vi "Teleop.vi"(10 "Match Info":T1={"Autonomous Elapsed Seconds"=0.0, "TeleOp Elapsed Seconds"=0.0, "Disabled Elapsed Seconds"=0.0, "Visited Autonomous"=FALSE, "Visited TeleOp"=FALSE, "Visited Disabled"=FALSE, "Autonomous Settings"={"Autonomous Style"=enum."Independent", "VI Refnum"=refnum}}, 11 "Call Context":T2) -> ()   [LabVIEW 2019]
doc: "This VI is called for each TeleOp packet received from the DS where the robot is not disabled. It is often used to read from the joysticks and update I/O or to update setpoints for timed control loops. It should complete and return within 20 milliseconds or it may miss DS packets."
uses:
  <vilib>/Rock Robotics/Network Tables/NT Write Numeric Array.vi
  Robot Global Data.vi
  <vilib>/Rock Robotics/Network Tables/NT Write Number.vi
  <vilib>/Rock Robotics/Network Tables/NT Write Variant.vi
  <vilib>/Rock Robotics/Network Tables/NT Write Boolean.vi
  <vilib>/Rock Robotics/Network Tables/NT Write Boolean Array.vi
  <vilib>/Rock Robotics/Network Tables/NT Write String.vi
  <vilib>/Rock Robotics/WPI/DriverStation/WPI_DriverStationMatch Info.ctl
  <vilib>/Rock Robotics/WPI/DriverStation/WPI_DriverStationDerivedRobotMode.ctl
panel:
  in  "Blue Cal":cluster{"R":dbl, "G":dbl, "B":dbl}={"R"=0.143, "G"=0.427, "B"=0.429} caption="Blue Calibration"
  in  "Green Cal":cluster{"R":dbl, "G":dbl, "B":dbl}={"R"=0.197, "G"=0.561, "B"=0.24} caption="Green Calibration"
  in  "Red Cal":cluster{"R":dbl, "G":dbl, "B":dbl}={"R"=0.561, "G"=0.323, "B"=0.114} caption="Red Calibration"
  in  "Yellow Cal":cluster{"R":dbl, "G":dbl, "B":dbl}={"R"=0.361, "G"=0.524, "B"=0.113} caption="Yellow Calibration"
  out "Matched Color Name":string
  out "Match Confidence":dbl
  out "Measured Color":cluster{"R":dbl, "G":dbl, "B":dbl}
  out "error out 2":errorcluster
  out "Proximity":u16(graph)
  out "Color":u32(colorbox)
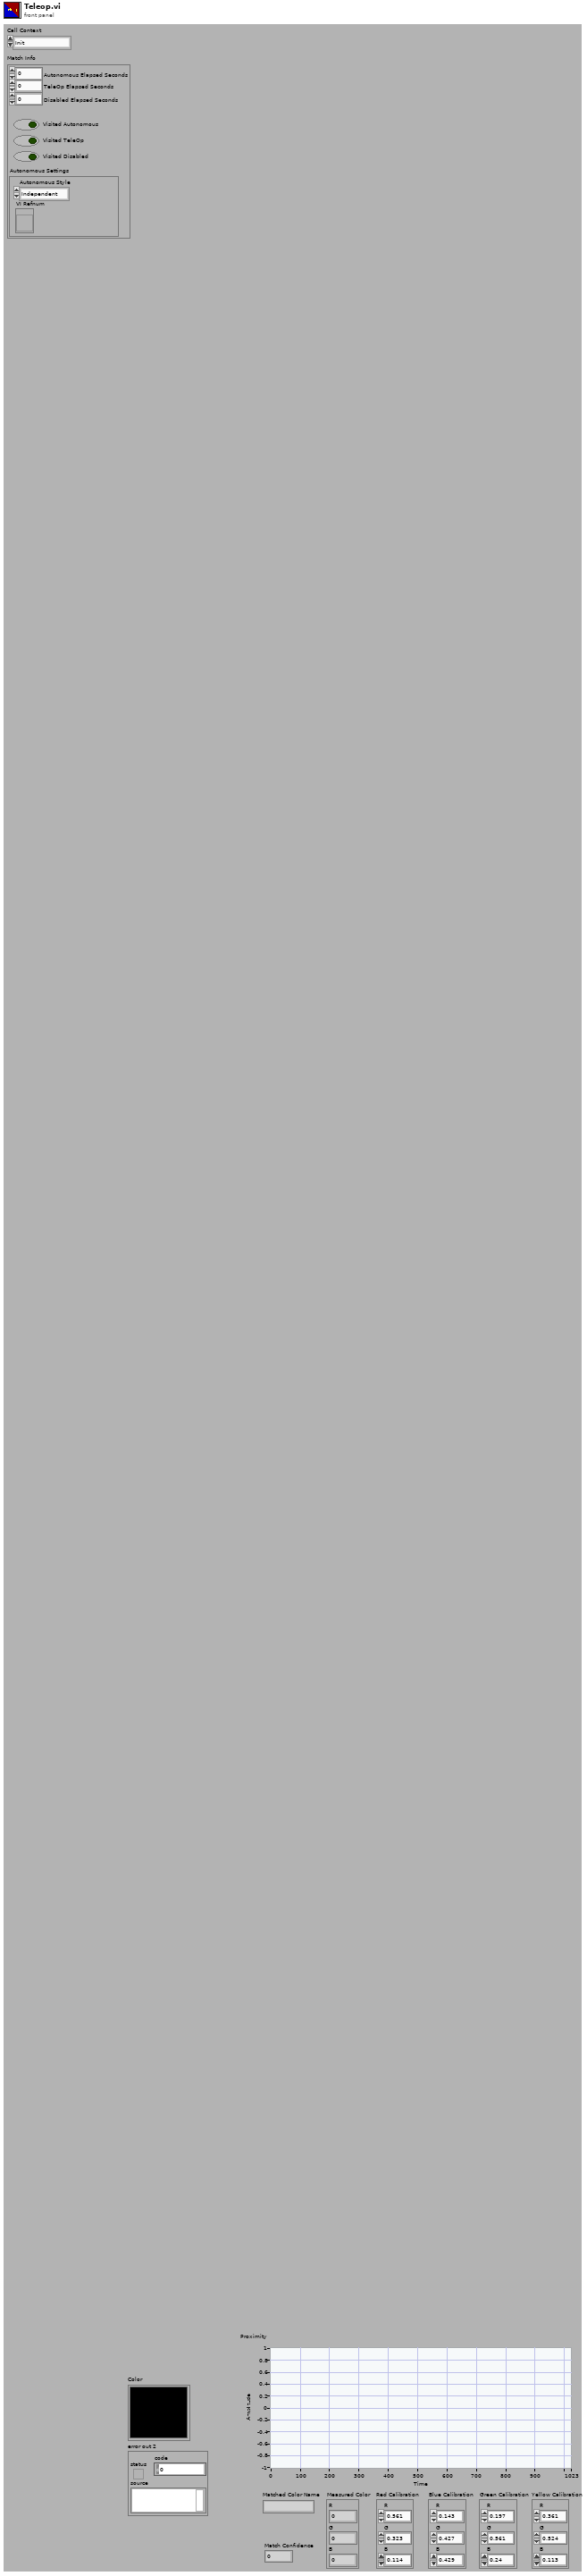
[diagram p1: front panel]
types:
  T1 = typedef "WPI_DriverStationMatch Info.ctl" = cluster{"Autonomous Elapsed Seconds":dbl, "TeleOp Elapsed Seconds":dbl, "Disabled Elapsed Seconds":dbl, "Visited Autonomous":bool, "Visited TeleOp":bool, "Visited Disabled":bool, "Autonomous Settings":cluster{"Autonomous Style":enum16{"Iterative", "Independent"}, "VI Refnum":refnum<vi>}}
  T2 = typedef "WPI_DriverStationDerivedRobotMode.ctl" = enum16{"Init", "Execute", "Stop"}
  T3 = typedef "WPI_RobotDriveDevRef.ctl" = cluster{"DevStatus":errorcluster, "Motors[]":T4[], "Square Inputs":bool, "Max Output":dbl}
  T4 = typedef "WPI_MotorControlDeviceRef.ctl" = cluster{"DeviceStatus":errorcluster, "Type":T5, "PWM":cluster{"PWM Channel":T6, "DeadBand":T7}, "CAN":cluster{"Device Number":u8, "SetOutput VI Ref":variant, "GetOutput VI Ref":variant, "Enable VI Ref":variant, "Disable VI Ref":variant, "Data":variant}, "Invert":bool, "DIO PWM":cluster{"PWM \"Enable\" Channel":T6, "DIOChannel":T8, "PWM Rate":dbl}}
  T5 = typedef "WPI_MotorControlType.ctl" = enum16{"PWM", "CAN", "DIO PWM"}
  T6 = typedef "FPGA_DIOPWMChannel.ctl" = enum8{"PWM 0", "PWM 1", "PWM 2", "PWM 3", "PWM 4", "PWM 5", "PWM 6", "PWM 7", "PWM 8", "PWM 9", "PWM MXP 0", "PWM MXP 1", "PWM MXP 2", "PWM MXP 3", "PWM MXP 4", "PWM MXP 5", "PWM MXP 6", "PWM MXP 7", "PWM MXP 8", "PWM MXP 9", "Invalid"}
  T7 = typedef "WPI_PWMDeadband.ctl" = cluster{"Name":string, "maxPositivePwm":i32, "minPositivePwm":i32, "centerPwm":i32, "maxNegativePwm":i32, "minNegativePwm":i32, "angularRange":u16}
  T8 = typedef "FPGA_DIOChannel.ctl" = enum8{"DIO 0", "DIO 1", "DIO 2", "DIO 3", "DIO 4", "DIO 5", "DIO 6", "DIO 7", "DIO 8", "DIO 9", "DIO MXP 0", "DIO MXP 1", "DIO MXP 2", "DIO MXP 3", "DIO MXP 4", "DIO MXP 5", "DIO MXP 6", "DIO MXP 7", "DIO MXP 8", "DIO MXP 9", "DIO MXP 10", "DIO MXP 11", "DIO MXP 12", "DIO MXP 13", "DIO MXP 14", "DIO MXP 15", "SPI Port CS1", "SPI Port CS2", "SPI Port CS3", "SPI Port MISO", "SPI Port MOSI", "Invalid"}
  T9 = typedef "WPI_JoystickDevRef.ctl" = cluster{"Device":T10}
  T10 = typedef "WPI_JoystickDeviceEnum.ctl" = enum16{"USB 0", "USB 1", "USB 2", "USB 3", "USB 4", "USB 5"}
  T11 = cluster{"JoystickDevRef":T9, "RobotDriveDevRef":T3}
  T12 = typedef "WPI_SwitchDevRef.ctl" = cluster{"DevStatus":errorcluster, "DIO Channel":T8, "CntIndex":T13, "Normally Closed":bool}
  T13 = typedef "FPGA_CounterCtrSystemIndex.ctl" = enum8{"Ctr 0", "Ctr 1", "Ctr 2", "Ctr 3", "Ctr 4", "Ctr 5", "Ctr 6", "Ctr 7", "Invalid"}
  T14 = typedef "Color Sensor V3 DevRef.ctl" = cluster{"I2CDevRef":T15}
  T15 = typedef "WPI_I2CDevRef.ctl" = cluster{"DevStatus":errorcluster, "Device Address":u8, "Handle":i32, "I2C Bus":T16}
  T16 = typedef "i2c_bus.ctl" = enum16{"I2C On-Board", "I2C MXP", "Invalid"}
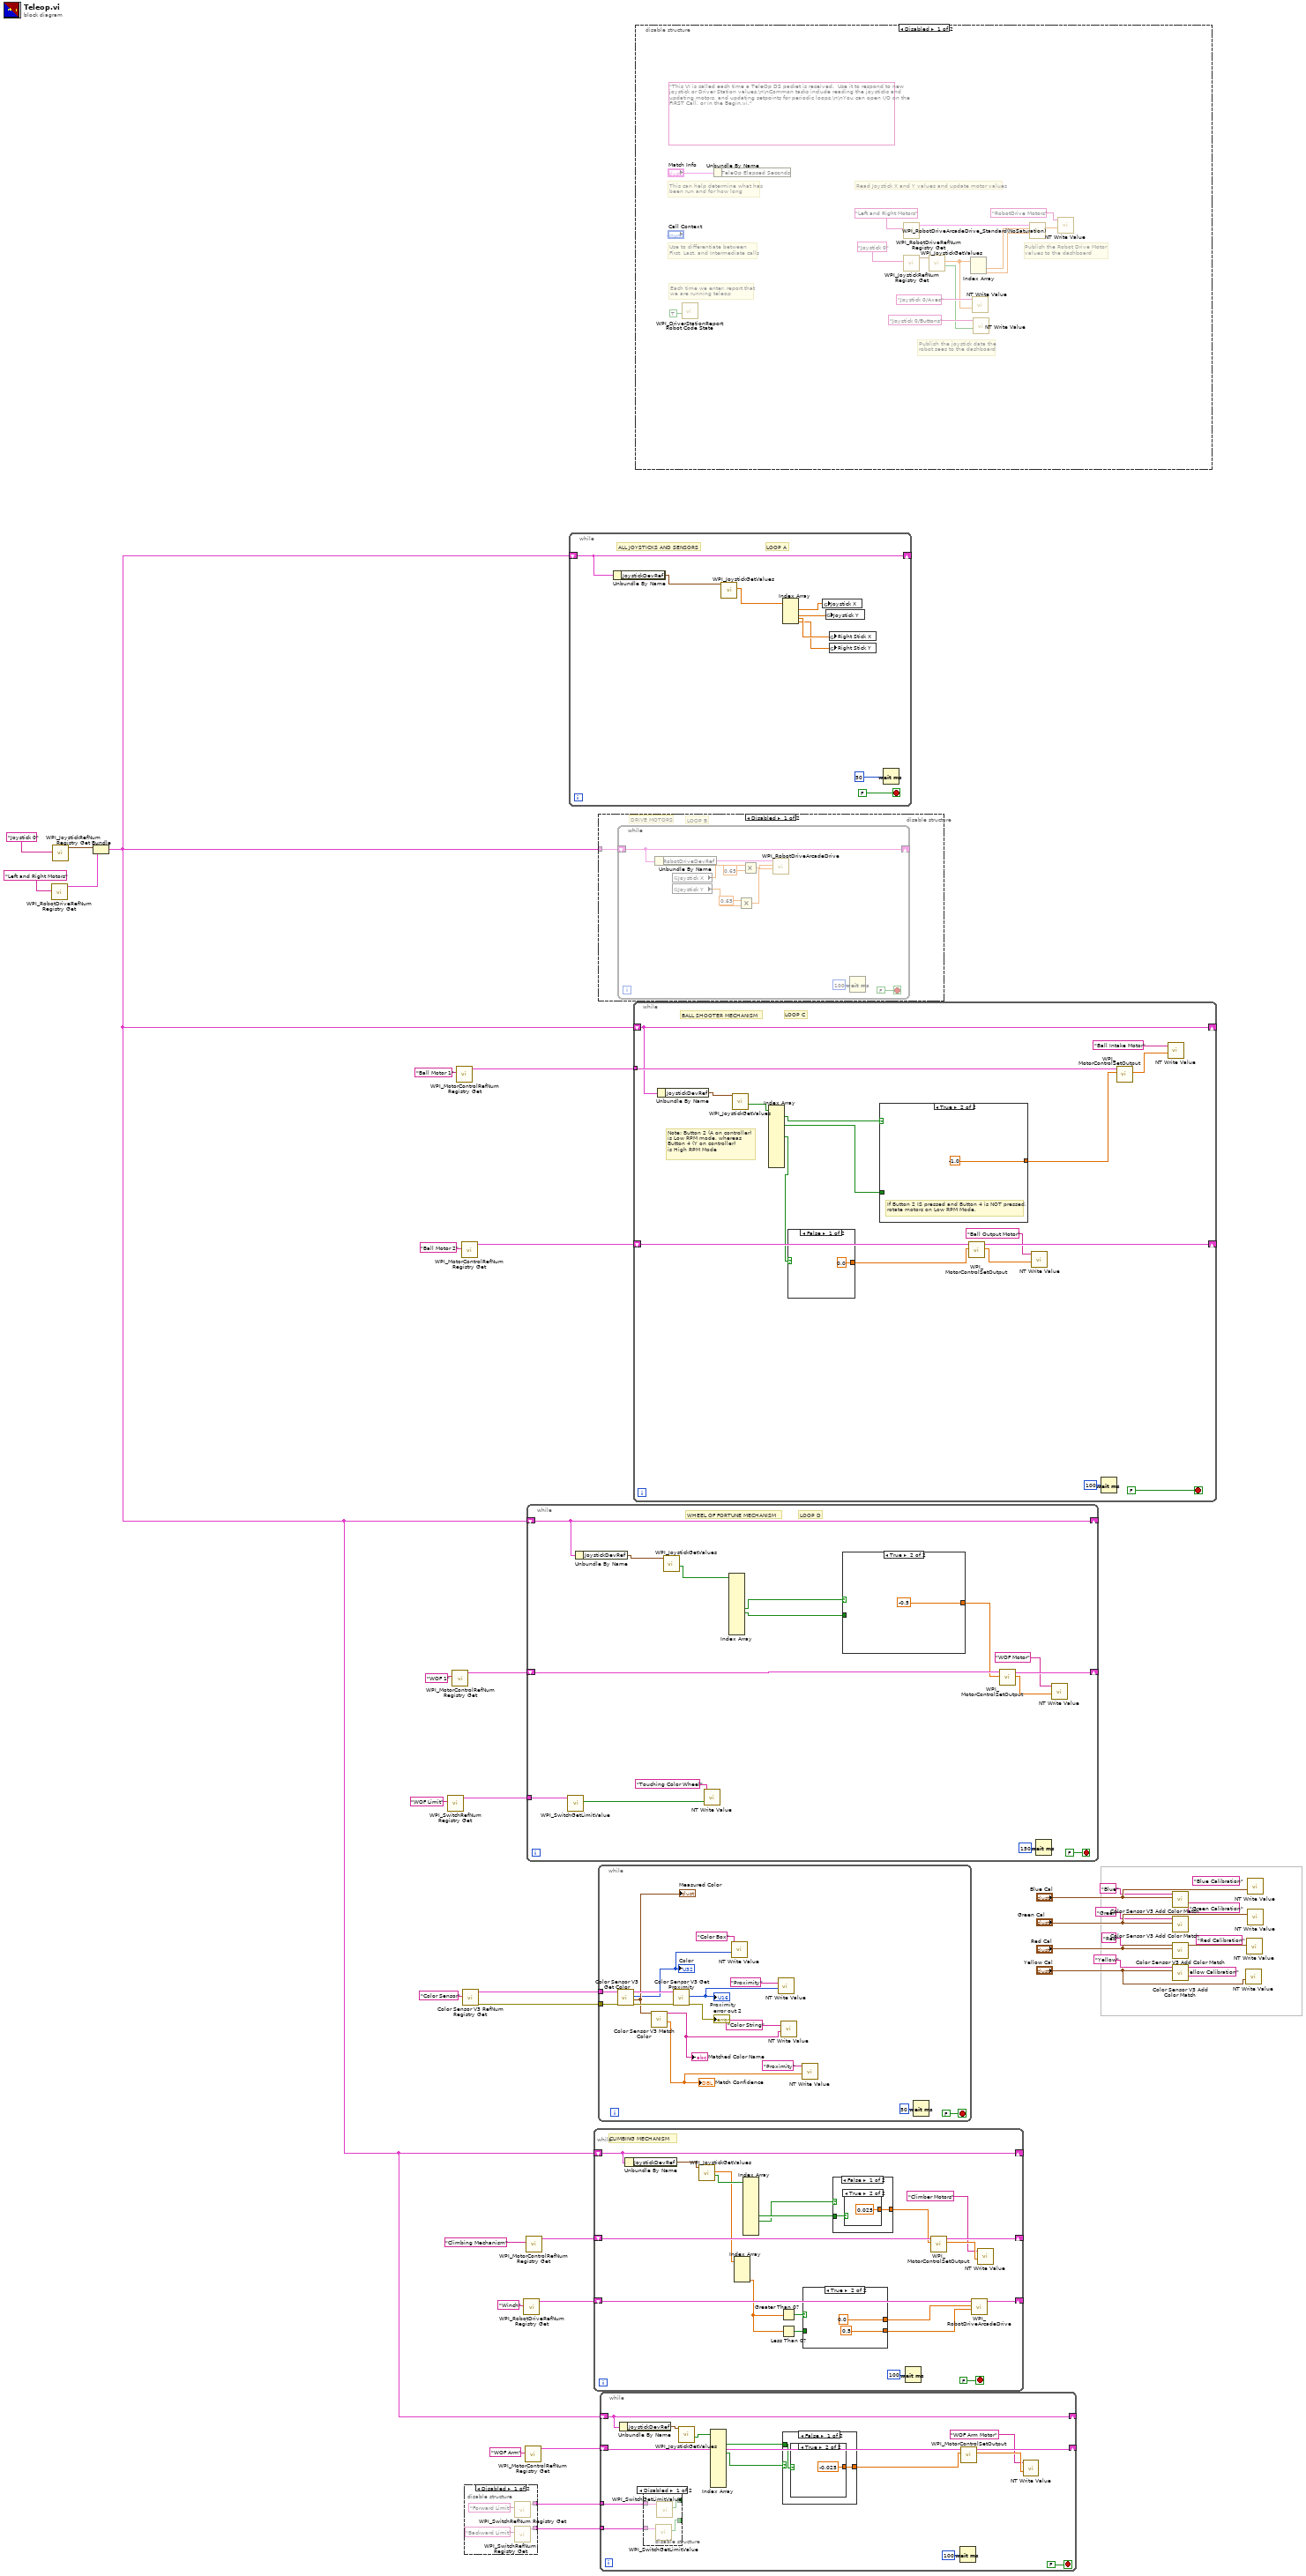
[diagram p0: block diagram]
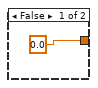
[diagram p3: hidden frame]
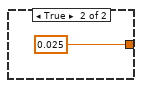
[diagram p4: hidden frame]
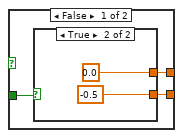
[diagram p6: hidden frame]
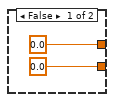
[diagram p7: hidden frame]
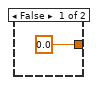
[diagram p8: hidden frame]
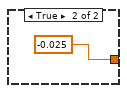
[diagram p9: hidden frame]
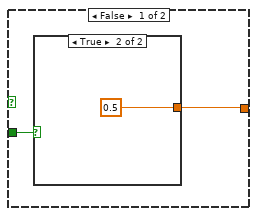
[diagram p12: hidden frame]
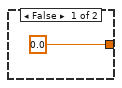
[diagram p13: hidden frame]
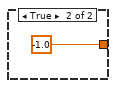
[diagram p14: hidden frame]
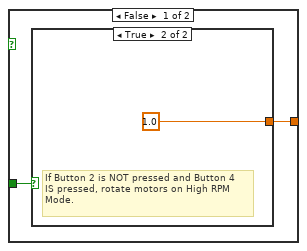
[diagram p15: hidden frame]
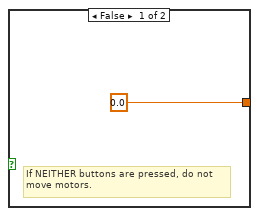
[diagram p16: hidden frame]
diagram:
  (unwired) "Yellow Calibration" ("Name")
  (unwired) "Red Calibration" ("Name")
  (unwired) "Green Calibration" ("Name")
  (unwired) "Blue Calibration" ("Name")
  n1 = call <vilib>:"WPI_RobotDriveRefNum Registry Get.vi"("refnum name"="Left and Right Motors") -> ("RobotDriveDevRef"=w29:T3)  [unwired: 1 in, 9 out]
  n2 = call <vilib>:"WPI_JoystickRefNum Registry Get.vi"("refnum name"="Joystick 0") -> ("JoystickDevRef"=w30:T9)  [unwired: 1 in, 9 out]
  n3 = Bundle("JoystickDevRef"=w30, "RobotDriveDevRef"=w29) -> (w5:T11)  [unwired: 1 out]
  n4 = call <vilib>:"WPI_SwitchRefNum Registry Get.vi"("refnum name"="WOF Limit") -> ("SwitchDevRef"=w10:T12)  [unwired: 9 in, 1 out]
  n5 = call <vilib>:"WPI_MotorControlRefNum Registry Get.vi"("refnum name"="WOF 1") -> ("MotorControlDevRef"=w25:T4)  [unwired: 9 in, 1 out]
  n6 = call <vilib>:"WPI_MotorControlRefNum Registry Get.vi"("refnum name"="Ball Motor 1") -> ("MotorControlDevRef"=w27:T4)  [unwired: 9 in, 1 out]
  n7 = call <vilib>:"WPI_MotorControlRefNum Registry Get.vi"("refnum name"="Ball Motor 2") -> ("MotorControlDevRef"=w12:T4)  [unwired: 9 in, 1 out]
  n8 = call <vilib>:"Color Sensor V3 RefNum Registry Get.vi"("refnum name"="Color Sensor") -> ("error out"=w15:errorcluster, "ColorSensorDevRef"=w16:T14)  [unwired: 9 in]
  n9 = disable-structure shown="Disabled" {
    disable-tunnel: [w34 _] -> w4
    disable-tunnel: [w33 _] -> w3
    frame Disabled {
      n10 = call <vilib>:"WPI_SwitchRefNum Registry Get.vi"("refnum name"="Forward Limit") -> ("SwitchDevRef"=w34:T12)  [unwired: 9 in, 1 out]
      n11 = call <vilib>:"WPI_SwitchRefNum Registry Get.vi"("refnum name"="Backward Limit") -> ("SwitchDevRef"=w33:T12)  [unwired: 9 in, 1 out]
    }
    frame Enabled {
    }
  }
  n12 = call <vilib>:"WPI_RobotDriveRefNum Registry Get.vi"("refnum name"="Winch") -> ("RobotDriveDevRef"=w2:T3)  [unwired: 9 in, 1 out]
  n13 = call <vilib>:"WPI_MotorControlRefNum Registry Get.vi"("refnum name"="WOF Arm") -> ("MotorControlDevRef"=w7:T4)  [unwired: 9 in, 1 out]
  n14 = call <vilib>:"WPI_MotorControlRefNum Registry Get.vi"("refnum name"="Climbing Mechanism") -> ("MotorControlDevRef"=w9:T4)  [unwired: 9 in, 1 out]
  n15 = while {
    shift-right: [w50] -> _
    shift-left: w5 -> [w50]
    shift-right: [w47] -> _
    shift-left: w25 -> [w48]
    tunnel: w10 -> [w44]
    stop <- FALSE stop-if-true
    # "LOOP D"
    # "WHEEL OF FORTUNE MECHANISM"
    n16 = call <vilib>:"WPI_SwitchGetLimitValue.vi"("SwitchDevRef"=w44) -> ("Switch Pressed"=w42:bool)  [unwired: 8 in, 2 out]
    n17 = Unbundle By Name(w50) -> ("JoystickDevRef"=w49:T9)
    n18 = call <vilib>:"WPI_JoystickGetValues.vi"("JoystickDevRef"=w49) -> ("Buttons"=w41:bool[])  [unwired: 6 in, 4 out]
    n19 = call-poly <vilib>:"NT Write Value.vi"("Boolean"=w42, "Name"="Touching Color Wheel") -> ()  [unwired: 9 in, 1 out]
    n20 = Index Array(array=w41) -> (element #7=w40:bool, element #8=w39:bool)  [unwired: 13 in, 11 out]
    n21 = case shown="True" w40 {
      tunnel: [w53 -0.5 ("Output")] -> w46
      tunnel: w39 -> [w52 _]
      frame False {
        n22 = case shown="True" w52 {
          tunnel: [0.0 ("Output") 0.5 ("Output")] -> w53
          frame False {
          }
          frame True {
          }
        }
      }
      frame True {
      }
    }
    n23 = call <vilib>:"WPI_MotorControlSetOutput.vi"("Output"=w46, "MotorControlDevRef"=w48) -> ("Motor Output"=w38:dbl, "MotorControlDevRef"=w47:T4)  [unwired: 7 in, 1 out]
    n24 = Wait (ms)(milliseconds to wait=u32 150) -> ()  [unwired: 1 out]
    n25 = call-poly <vilib>:"NT Write Value.vi"("Numeric"=w38, "Name"="WOF Motor") -> ()  [unwired: 9 in, 1 out]
  }
  n26 = while {
    shift-right: [w64] -> _
    shift-left: w5 -> [w64]
    stop <- FALSE stop-if-true
    # "LOOP A"
    # "ALL JOYSTICKS AND SENSORS"
    n27 = Unbundle By Name(w64) -> ("JoystickDevRef"=w63:T9)
    n28 = call <vilib>:"WPI_JoystickGetValues.vi"("JoystickDevRef"=w63) -> ("Axes"=w62:dbl[])  [unwired: 6 in, 4 out]
    n29 = Index Array(array=w62) -> (element #1=w60:dbl, element #2=w61:dbl, element #3=w58:dbl, element #4=w57:dbl)  [unwired: 4 in]
    n30 = global write "Robot Global Data.vi" "Joystick X"(w60) -> ()
    n31 = global write "Robot Global Data.vi" "Joystick Y"(w61) -> ()
    n32 = global write "Robot Global Data.vi" "Right Stick X"(w58) -> ()
    n33 = global write "Robot Global Data.vi" "Right Stick Y"(w57) -> ()
    n34 = Wait (ms)(milliseconds to wait=u32 50) -> ()  [unwired: 1 out]
  }
  n35 = while {
    shift-right: [w74] -> _
    shift-left: w5 -> [w74]
    shift-right: [w83] -> _
    shift-left: w9 -> [w82]
    shift-right: [w73] -> _
    shift-left: w2 -> [w72]
    stop <- FALSE stop-if-true
    # "CLIMBING MECHANISM"
    n36 = Unbundle By Name(w74) -> ("JoystickDevRef"=w85:T9)
    n37 = call <vilib>:"WPI_JoystickGetValues.vi"("JoystickDevRef"=w85) -> ("Buttons"=w84:bool[], "Axes"=w71:dbl[])  [unwired: 6 in, 3 out]
    n38 = Index Array(array=w71) -> (element #4=w68:dbl)  [unwired: 4 in, 3 out]
    n39 = Index Array(array=w84) -> (element #9=w78:bool, element #10=w79:bool)  [unwired: 12 in, 10 out]
    n40 = Greater Than 0?(x=w68) -> (x > 0?=w70:bool)
    n41 = Less Than 0?(x=w68) -> (x < 0?=w69:bool)
    n42 = case shown="True" w70 {
      tunnel: w69 -> [w88 _]
      tunnel: [w87 0.0 ("X axis value")] -> w67
      tunnel: [w86 0.5 ("Y axis value")] -> w66
      frame False {
        n43 = case shown="True" w88 {
          tunnel: [0.0 ("X axis value") 0.0 ("X axis value")] -> w87
          tunnel: [0.0 ("Y axis value") -0.5 ("Y axis value")] -> w86
          frame False {
          }
          frame True {
          }
        }
      }
      frame True {
      }
    }
    n44 = case shown="False" w78 {
      tunnel: [w96 -0.025 ("Output")] -> w80
      tunnel: w79 -> [w95 _]
      frame False {
        n45 = case shown="True" w95 {
          tunnel: [0.0 ("Output") 0.025 ("Output")] -> w96
          frame False {
          }
          frame True {
          }
        }
      }
      frame True {
      }
    }
    n46 = Wait (ms)(milliseconds to wait=u32 100) -> ()  [unwired: 1 out]
    n47 = call <vilib>:"WPI_MotorControlSetOutput.vi"("Output"=w80, "MotorControlDevRef"=w82) -> ("Motor Output"=w77:dbl, "MotorControlDevRef"=w83:T4)  [unwired: 7 in, 1 out]
    n48 = call-poly <vilib>:"WPI_RobotDriveArcadeDrive.vi"("Y axis value"=w66, "X axis value"=w67, "RobotDriveDevRef"=w72) -> ("RobotDriveDevRef"=w73:T3)  [unwired: 6 in, 2 out]
    n49 = call-poly <vilib>:"NT Write Value.vi"("Numeric"=w77, "Name"="Climber Motors") -> ()  [unwired: 9 in, 1 out]
  }
  n50 = disable-structure shown="Disabled" {
    disable-tunnel: w5 -> [w100 _]
    frame Disabled {
      # "LOOP B"
      # "DRIVE MOTORS"
      n51 = while {
        shift-right: [w108] -> _
        shift-left: w100 -> [w108]
        stop <- FALSE stop-if-true
        n52 = Unbundle By Name(w108) -> ("RobotDriveDevRef"=w107:T3)
        n53 = global read "Robot Global Data.vi" "Joystick X"() -> (w105:dbl)
        n54 = global read "Robot Global Data.vi" "Joystick Y"() -> (w106:dbl)
        n55 = Multiply(x=0.65, y=w106) -> (x*y=w102:dbl)
        n56 = Multiply(x=w105, y=0.65) -> (x*y=w101:dbl)
        n57 = call-poly <vilib>:"WPI_RobotDriveArcadeDrive.vi"("Y axis value"=w102, "X axis value"=w101, "RobotDriveDevRef"=w107) -> ()  [unwired: 6 in, 3 out]
        n58 = Wait (ms)(milliseconds to wait=u32 100) -> ()  [unwired: 1 out]
      }
    }
    frame Enabled {
    }
  }
  n59 = while {
    tunnel: w16 -> [w112]
    tunnel: w15 -> [w111]
    stop <- FALSE stop-if-true
    n60 = call <vilib>:"Color Sensor V3 Get Color.vi"("error in (no error)"=w111, "ColorSensorDevRef"=w112) -> ("error out"=w126:errorcluster, "Normalized Color"=w123:cluster{"R":dbl, "G":dbl, "B":dbl}, "Color"=w120:u32, "ColorSensorDevRef out"=w125:T14)  [unwired: 6 in]
    "Color" <- w120
    "Measured Color" <- w123
    n61 = call <vilib>:"Color Sensor V3 Match Color.vi"("Measured Color"=w123) -> ("Confidence"=w116:dbl, "Matched Color Name"=w114:string)  [unwired: 8 in, 1 out]
    "Match Confidence" <- w116
    "Matched Color Name" <- w114
    n62 = call <vilib>:"Color Sensor V3 Get Proximity.vi"("error in (no error)"=w126, "ColorSensorDevRef"=w125) -> ("error out"=→"error out 2":errorcluster, "Proximity"=w118:u16)  [unwired: 7 in, 1 out]
    "Proximity" <- w118
    n63 = call-poly <vilib>:"NT Write Value.vi"("Numeric"=w120, "Name"="Color Box") -> ()  [unwired: 9 in, 1 out]
    n64 = call-poly <vilib>:"NT Write Value.vi"("Numeric"=w118, "Name"="Proximity") -> ()  [unwired: 9 in, 1 out]
    n65 = call-poly <vilib>:"NT Write Value.vi"("String"=w114, "Name"="Color String") -> ()  [unwired: 9 in, 1 out]
    n66 = call-poly <vilib>:"NT Write Value.vi"("Numeric"=w116, "Name"="Proximity") -> ()  [unwired: 9 in, 1 out]
    n67 = Wait (ms)(milliseconds to wait=u32 50) -> ()  [unwired: 1 out]
  }
  n68 = while {
    shift-right: [w139] -> _
    shift-left: w7 -> [w138]
    shift-right: [w136] -> _
    shift-left: w5 -> [w136]
    tunnel: w4 -> [w134]
    tunnel: w3 -> [w133]
    stop <- FALSE stop-if-true
    n69 = Unbundle By Name(w136) -> ("JoystickDevRef"=w135:T9)
    n70 = disable-structure shown="Disabled" {
      disable-tunnel: w134 -> [w149 _]
      disable-tunnel: w133 -> [w148 _]
      disable-tunnel: [w147 _] -> _
      disable-tunnel: [w146 _] -> _
      frame Disabled {
        n71 = call <vilib>:"WPI_SwitchGetLimitValue.vi"("SwitchDevRef"=w148) -> ("Switch Pressed"=w146:bool)  [unwired: 8 in, 2 out]
        n72 = call <vilib>:"WPI_SwitchGetLimitValue.vi"("SwitchDevRef"=w149) -> ("Switch Pressed"=w147:bool)  [unwired: 8 in, 2 out]
      }
      frame Enabled {
      }
    }
    n73 = call <vilib>:"WPI_JoystickGetValues.vi"("JoystickDevRef"=w135) -> ("Buttons"=w137:bool[])  [unwired: 6 in, 4 out]
    n74 = Index Array(array=w137) -> (element #2=w130:bool, element #4=w132:bool)  [unwired: 12 in, 10 out]
    n75 = case shown="False" w132 {
      tunnel: [w141 0.025 ("Output")] -> w131
      tunnel: w130 -> [w142 _]
      frame False {
        n76 = case shown="True" w142 {
          tunnel: [0.0 ("Output") -0.025 ("Output")] -> w141
          frame False {
          }
          frame True {
          }
        }
      }
      frame True {
      }
    }
    n77 = Wait (ms)(milliseconds to wait=u32 100) -> ()  [unwired: 1 out]
    n78 = call <vilib>:"WPI_MotorControlSetOutput.vi"("Output"=w131, "MotorControlDevRef"=w138) -> ("Motor Output"=w129:dbl, "MotorControlDevRef"=w139:T4)  [unwired: 7 in, 1 out]
    n79 = call-poly <vilib>:"NT Write Value.vi"("Numeric"=w129, "Name"="WOF Arm Motor") -> ()  [unwired: 9 in, 1 out]
  }
  n80 = while {
    shift-right: [w160] -> _
    shift-left: w5 -> [w160]
    tunnel: w27 -> [w164]
    shift-right: [w158] -> _
    shift-left: w12 -> [w159]
    stop <- FALSE stop-if-true
    # "LOOP C"
    # "Note: Button 2 (A on controller) \nis Low RPM mode, whereas \nButton 4 (Y on controller)\nis High RPM Mode"
    # "BALL SHOOTER MECHANISM"
    n81 = Unbundle By Name(w160) -> ("JoystickDevRef"=w162:T9)
    n82 = call <vilib>:"WPI_JoystickGetValues.vi"("JoystickDevRef"=w162) -> ("Buttons"=w161:bool[])  [unwired: 6 in, 4 out]
    n83 = Index Array(array=w161) -> (element #1=w157:bool, element #3=w156:bool, element #6=w154:bool)  [unwired: 13 in, 10 out]
    n84 = case shown="False" w154 {
      tunnel: [0.0 ("Output") -1.0 ("Output")] -> w155
      frame False {
      }
      frame True {
      }
    }
    n85 = case shown="True" w157 {
      tunnel: [w170 -1.0 ("Output")] -> w163
      tunnel: w156 -> [w169 _]
      frame False {
        n86 = case shown="True" w169 {
          tunnel: [0.0 ("Output") 1.0 ("Output")] -> w170
          frame False {
            # "If NEITHER buttons are pressed, do not\nmove motors."
          }
          frame True {
            # "If Button 2 is NOT pressed and Button 4\nIS pressed, rotate motors on High RPM\nMode."
          }
        }
      }
      frame True {
        # "If Button 2 IS pressed and Button 4 is NOT pressed,\nrotate motors on Low RPM Mode."
      }
    }
    n87 = call <vilib>:"WPI_MotorControlSetOutput.vi"("Output"=w155, "MotorControlDevRef"=w159) -> ("Motor Output"=w151:dbl, "MotorControlDevRef"=w158:T4)  [unwired: 7 in, 1 out]
    n88 = call-poly <vilib>:"NT Write Value.vi"("Numeric"=w151, "Name"="Ball Output Motor") -> ()  [unwired: 9 in, 1 out]
    n89 = Wait (ms)(milliseconds to wait=u32 100) -> ()  [unwired: 1 out]
    n90 = call <vilib>:"WPI_MotorControlSetOutput.vi"("Output"=w163, "MotorControlDevRef"=w164) -> ("Motor Output"=w153:dbl)  [unwired: 7 in, 2 out]
    n91 = call-poly <vilib>:"NT Write Value.vi"("Numeric"=w153, "Name"="Ball Intake Motor") -> ()  [unwired: 9 in, 1 out]
  }
  n92 = disable-structure shown="Disabled" {
    frame Disabled {
      (unwired) "This VI is called each time a TeleOp DS packet is received.  Use it to respond to new joystick or Driver Station values.\n\nCommon tasks include reading the joysticks and updating motors, and updating setpoints for periodic loops.\n\nYou can open I/O on the FIRST Call, or in the Begin.vi."
      # "Publish the Robot Drive Motor\nvalues to the dashboard"
      # "Publish the joystick data the\nrobot sees to the dashboard"
      # "Each time we enter, report that\nwe are running teleop"
      # "Use to differentiate between\nFirst, Last, and Intermediate calls"
      # "This can help determine what has\nbeen run and for how long"
      # "Read Joystick X and Y values and update motor values"
      n93 = call <vilib>:"WPI_DriverStationReport Robot Code State.vi"("TeleOp"=TRUE ("Autonomous")) -> ()  [unwired: 10 in, 1 out]
      n94 = Unbundle By Name("Match Info") -> ()  [unwired: 1 out]
      n95 = call <vilib>:"WPI_RobotDriveRefNum Registry Get.vi"("refnum name"="Left and Right Motors") -> ("RobotDriveDevRef"=w185:T3)  [unwired: 1 in, 9 out]
      n96 = call <vilib>:"WPI_JoystickRefNum Registry Get.vi"("refnum name"="Joystick 0") -> ("JoystickDevRef"=w182:T9)  [unwired: 1 in, 9 out]
      n97 = call <vilib>:"WPI_JoystickGetValues.vi"("JoystickDevRef"=w182) -> ("Buttons"=w176:bool[], "Axes"=w177:dbl[])  [unwired: 6 in, 3 out]
      n98 = Index Array(array=w177) -> (element #1=w184:dbl, element #2=w180:dbl)  [unwired: 2 in]
      n99 = call-poly <vilib>:"NT Write Value.vi"("Numeric Array"=w177, "Name"="Joystick 0/Axes") -> ()  [unwired: 9 in, 1 out]
      n100 = call-poly <vilib>:"NT Write Value.vi"("Boolean Array"=w176, "Name"="Joystick 0/Buttons") -> ()  [unwired: 9 in, 1 out]
      n101 = call <vilib>:"WPI_RobotDriveArcadeDrive_Standard(NoSaturation).vi"("Y axis value"=w180, "X axis value"=w184, "RobotDriveDevRef"=w185) -> ("Motor Values"=w175:dbl[])  [unwired: 1 in, 7 out]
      n102 = call-poly <vilib>:"NT Write Value.vi"("Numeric Array"=w175, "Name"="RobotDrive Motors") -> ()  [unwired: 9 in, 1 out]
    }
    frame Enabled {
    }
  }
  n103 = call <vilib>:"Color Sensor V3 Add Color Match.vi"("Color"="Blue Cal", "Name"="Blue") -> ()  [unwired: 10 in]
  n104 = call <vilib>:"Color Sensor V3 Add Color Match.vi"("Color"="Green Cal", "Name"="Green") -> ()  [unwired: 10 in]
  n105 = call <vilib>:"Color Sensor V3 Add Color Match.vi"("Color"="Red Cal", "Name"="Red") -> ()  [unwired: 10 in]
  n106 = call <vilib>:"Color Sensor V3 Add Color Match.vi"("Color"="Yellow Cal", "Name"="Yellow") -> ()  [unwired: 10 in]
  n107 = call-poly <vilib>:"NT Write Value.vi"("Variant"="Yellow Cal") -> ()  [unwired: 10 in, 1 out]
  n108 = call-poly <vilib>:"NT Write Value.vi"("Variant"="Red Cal") -> ()  [unwired: 10 in, 1 out]
  n109 = call-poly <vilib>:"NT Write Value.vi"("Variant"="Blue Cal") -> ()  [unwired: 10 in, 1 out]
  n110 = call-poly <vilib>:"NT Write Value.vi"("Variant"="Green Cal") -> ()  [unwired: 10 in, 1 out]
